vi "ArmControl.vi"(0 "ButtonArray":bool[](array[boolean])) -> ()   [LabVIEW 2018]
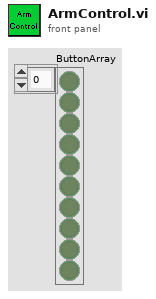
[diagram p1: front panel]
types:
  T1 = typedef "WPI_MotorControlDeviceRef.ctl" = cluster{"DeviceStatus":errorcluster, "Type":T2, "PWM":cluster{"PWM Channel":T3, "DeadBand":T4}, "CAN":cluster{"Device Number":u8, "SetOutput VI Ref":variant, "GetOutput VI Ref":variant, "Enable VI Ref":variant, "Disable VI Ref":variant, "Data":variant}, "Invert":bool, "DIO PWM":cluster{"PWM \"Enable\" Channel":T3, "DIOChannel":T5, "PWM Rate":dbl}}
  T2 = typedef "WPI_MotorControlType.ctl" = enum16{"PWM", "CAN", "DIO PWM"}
  T3 = typedef "FPGA_DIOPWMChannel.ctl" = enum8{"PWM 0", "PWM 1", "PWM 2", "PWM 3", "PWM 4", "PWM 5", "PWM 6", "PWM 7", "PWM 8", "PWM 9", "PWM MXP 0", "PWM MXP 1", "PWM MXP 2", "PWM MXP 3", "PWM MXP 4", "PWM MXP 5", "PWM MXP 6", "PWM MXP 7", "PWM MXP 8", "PWM MXP 9", "Invalid"}
  T4 = typedef "WPI_PWMDeadband.ctl" = cluster{"Name":string, "maxPositivePwm":i32, "minPositivePwm":i32, "centerPwm":i32, "maxNegativePwm":i32, "minNegativePwm":i32, "angularRange":u16}
  T5 = typedef "FPGA_DIOChannel.ctl" = enum8{"DIO 0", "DIO 1", "DIO 2", "DIO 3", "DIO 4", "DIO 5", "DIO 6", "DIO 7", "DIO 8", "DIO 9", "DIO MXP 0", "DIO MXP 1", "DIO MXP 2", "DIO MXP 3", "DIO MXP 4", "DIO MXP 5", "DIO MXP 6", "DIO MXP 7", "DIO MXP 8", "DIO MXP 9", "DIO MXP 10", "DIO MXP 11", "DIO MXP 12", "DIO MXP 13", "DIO MXP 14", "DIO MXP 15", "SPI Port CS1", "SPI Port CS2", "SPI Port CS3", "SPI Port MISO", "SPI Port MOSI", "Invalid"}
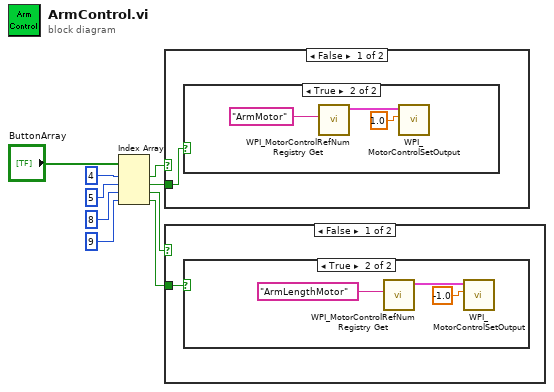
[diagram p0: block diagram]
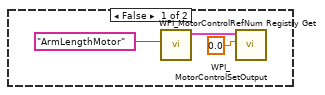
[diagram p2: hidden frame]
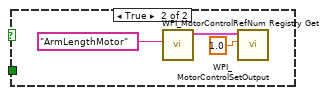
[diagram p3: hidden frame]
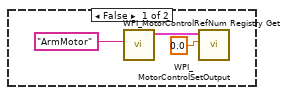
[diagram p4: hidden frame]
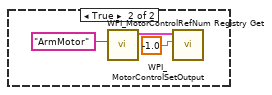
[diagram p5: hidden frame]
diagram:
  n1 = Index Array(array="ButtonArray", index #1=4 ("index"), index #2=5 ("index"), index #3=8 ("index"), index #4=9 ("index")) -> (element #1=w8:bool, element #2=w7:bool, element #3=w3:bool, element #4=w4:bool)
  n2 = case shown="False" w8 {
    tunnel: w7 -> [w10 _]
    frame False {
      n3 = case shown="True" w10 {
        frame False {
          n4 = call <vilib>:"WPI_MotorControlRefNum Registry Get.vi"("refnum name"="ArmMotor") -> ("MotorControlDevRef"=w13:T1)  [unwired: 9 in, 1 out]
          n5 = call <vilib>:"WPI_MotorControlSetOutput.vi"("Output"=0.0, "MotorControlDevRef"=w13) -> ()  [unwired: 7 in, 3 out]
        }
        frame True {
          n6 = call <vilib>:"WPI_MotorControlRefNum Registry Get.vi"("refnum name"="ArmMotor") -> ("MotorControlDevRef"=w16:T1)  [unwired: 9 in, 1 out]
          n7 = call <vilib>:"WPI_MotorControlSetOutput.vi"("Output"=1.0, "MotorControlDevRef"=w16) -> ()  [unwired: 7 in, 3 out]
        }
      }
    }
    frame True {
      n8 = call <vilib>:"WPI_MotorControlRefNum Registry Get.vi"("refnum name"="ArmMotor") -> ("MotorControlDevRef"=w19:T1)  [unwired: 9 in, 1 out]
      n9 = call <vilib>:"WPI_MotorControlSetOutput.vi"("Output"=-1.0, "MotorControlDevRef"=w19) -> ()  [unwired: 7 in, 3 out]
    }
  }
  n10 = case shown="False" w3 {
    tunnel: w4 -> [w20 _]
    frame False {
      n11 = case shown="True" w20 {
        frame False {
          n12 = call <vilib>:"WPI_MotorControlRefNum Registry Get.vi"("refnum name"="ArmLengthMotor") -> ("MotorControlDevRef"=w23:T1)  [unwired: 9 in, 1 out]
          n13 = call <vilib>:"WPI_MotorControlSetOutput.vi"("Output"=0.0, "MotorControlDevRef"=w23) -> ()  [unwired: 7 in, 3 out]
        }
        frame True {
          n14 = call <vilib>:"WPI_MotorControlRefNum Registry Get.vi"("refnum name"="ArmLengthMotor") -> ("MotorControlDevRef"=w26:T1)  [unwired: 9 in, 1 out]
          n15 = call <vilib>:"WPI_MotorControlSetOutput.vi"("Output"=-1.0, "MotorControlDevRef"=w26) -> ()  [unwired: 7 in, 3 out]
        }
      }
    }
    frame True {
      n16 = call <vilib>:"WPI_MotorControlRefNum Registry Get.vi"("refnum name"="ArmLengthMotor") -> ("MotorControlDevRef"=w29:T1)  [unwired: 9 in, 1 out]
      n17 = call <vilib>:"WPI_MotorControlSetOutput.vi"("Output"=1.0, "MotorControlDevRef"=w29) -> ()  [unwired: 7 in, 3 out]
    }
  }
